vi "Write VeriSTAND Channel Info.vi"(7 "Supported in CD":bool, 8 "error in (no error)":errorcluster, 9 "VeriSTAND Reference":T1=18446744073709551615 format="%.0x", 10 "Exist in VeriSTAND":bool, 11 "ChannelVS in":refnum<class "ChannelVS.lvclass">) -> (0 "error out":errorcluster, 3 "ChannelVS out":refnum<class "ChannelVS.lvclass">)   [LabVIEW 2020, in "Shared Variables CD 2.0 Configuration.lvlib" / "ChannelVS.lvclass"]
uses:
  ChannelVS.lvclass
  <vilib>/NI VeriStand/Custom Device API/Custom Device Item Ref.ctl
  <vilib>/NI VeriStand/Custom Device API/Custom Device API.lvlib
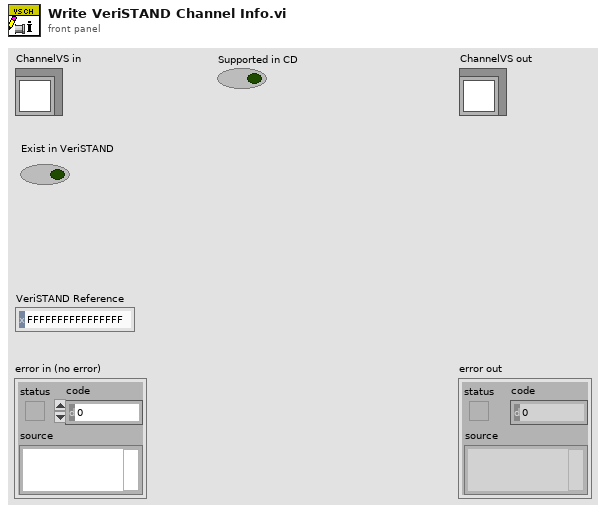
[diagram p1: front panel]
types:
  T1 = typedef "Custom Device API.lvlib/Custom Device Item Ref.ctl" = u64
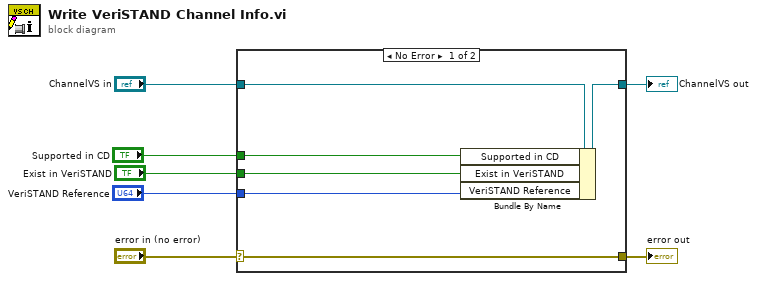
[diagram p0: block diagram]
diagram:
  n1 = case shown="No Error" "error in (no error)" {
    selector: "error in (no error)" -> [w13 w14]
    tunnel: [w13 w14] -> w6
    tunnel: [w11 w15] -> w4
    tunnel: "ChannelVS in" -> [w12 w15]
    tunnel: "Exist in VeriSTAND" -> [w10 _]
    tunnel: "VeriSTAND Reference" -> [w9 _]
    tunnel: "Supported in CD" -> [w8 _]
    frame No Error {
      n2 = Bundle By Name(cluster=w12, "Supported in CD"=w8, "Exist in VeriSTAND"=w10, "VeriSTAND Reference"=w9) -> (w11:refnum<class "ChannelVS.lvclass">)
    }
    frame Error {
    }
  }
  "error out" <- w6
  "ChannelVS out" <- w4
